vi "Player Info.vi"(8 "Victory Speech":string="Let Chaos Rule", 9 "Name":string="Spread", 11 "Spread in":refnum<class "Spread.lvclass">) -> (3 "Spread out":refnum<class "Spread.lvclass">)   [LabVIEW 2015, in "Spread.lvclass"]
uses:
  Spread.lvclass
  Square/Square.lvclass
panel:
  # "Set default values for these two string controls"
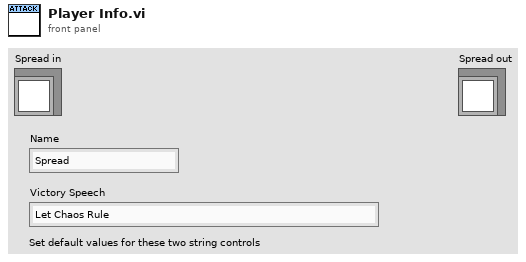
[diagram p1: front panel]
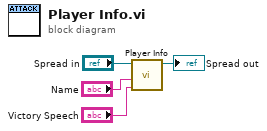
[diagram p0: block diagram]
diagram:
  n1 = call-parent "Player Info.vi"("Victory Speech"="Victory Speech", "Name"="Name", "Square in"="Spread in") -> ("Square out"=→"Spread out":refnum<class "Spread.lvclass">)  [unwired: 8 in]
